vi "Threshold A by 5% B.vi"(10 "array B":dbl[](array[numeric]), 11 "array A":dbl[](array[numeric])) -> (1 "Where array B = 100% of array A":dbl, 2 "threshold difference":dbl, 3 "Where array B = 95% of array A":dbl, 4 "index of 95% of array A":dbl)   [LabVIEW 2017, in "Processing.lvlib"]
uses:
  Processing.lvlib
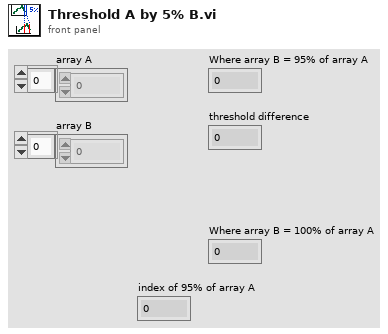
[diagram p1: front panel]
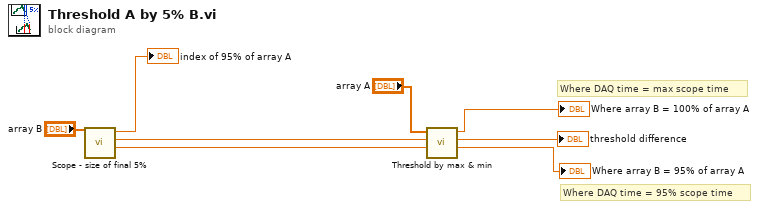
[diagram p0: block diagram]
diagram:
  # "Where DAQ time = max scope time"
  # "Where DAQ time = 95% scope time"
  n1 = call "Scope - size of final 5%.vi"("Scope time axis"="array B") -> ("95% of scope time"=w7:dbl, "max scope time"=w6:dbl, "Size of final 5% of scope time"=→"index of 95% of array A":dbl)  [unwired: 8 in]
  n2 = call "Threshold by max & min.vi"("min"=w7, "max"=w6, "array"="array A") -> ("index of min value"=→"Where array B = 95% of array A":dbl, "index of max - index of min"=→"threshold difference":dbl, "index of max value"=→"Where array B = 100% of array A":dbl)  [unwired: 6 in]
